vi "Code Point Substring.vi"(5 "End":i32, 7 "Start":i32, 11 "Constructor String Parser":T1) -> (3 "Substring":string)   [LabVIEW 2020, in "Stream.lvlib" / "URLPattern.lvclass"]
uses:
  URLPattern.lvclass
  Token Type.ctl
  Token.ctl
  URL Pattern Init.ctl
  Parser State.ctl
  Constructor String Parser.ctl
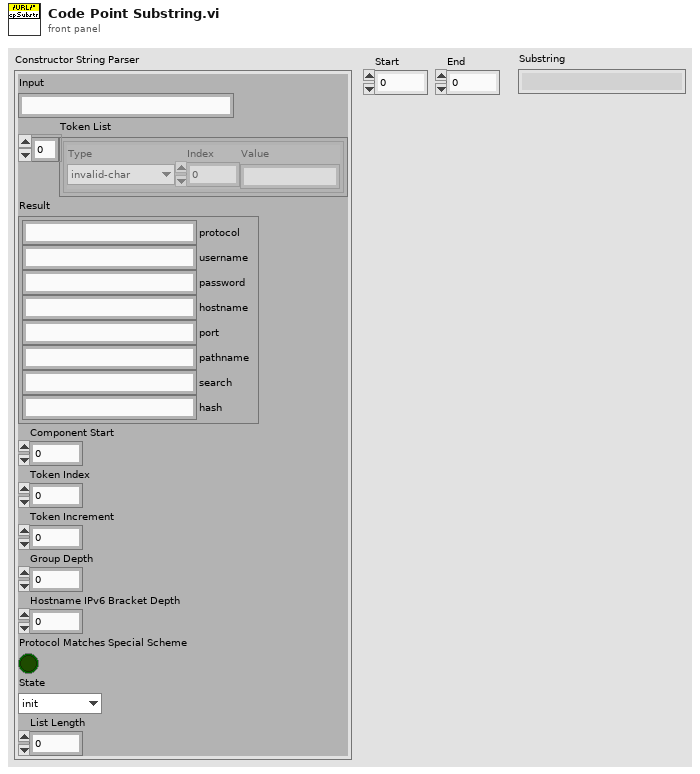
[diagram p1: front panel]
types:
  T1 = typedef "Stream.lvlib/URLPattern.lvclass/Constructor String Parser.ctl" = cluster{"Input":string, "Token List":T2[], "Result":T4, "Component Start":i32, "Token Index":i32, "Token Increment":i32, "Group Depth":i32, "Hostname IPv6 Bracket Depth":i32, "Protocol Matches Special Scheme":bool, "State":T5, "List Length":i32}
  T2 = typedef "Stream.lvlib/URLPattern.lvclass/Token.ctl" = cluster{"Type":T3, "Index":i32, "Value":string}
  T3 = typedef "Stream.lvlib/URLPattern.lvclass/Token Type.ctl" = enum16{"invalid-char", "open", "close", "regexp", "name", "char", "escaped-char", "other-modifier", "asterisk", "end"}
  T4 = typedef "Stream.lvlib/URLPattern.lvclass/URL Pattern Init.ctl" = cluster{"protocol":string, "username":string, "password":string, "hostname":string, "port":string, "pathname":string, "search":string, "hash":string}
  T5 = typedef "Stream.lvlib/URLPattern.lvclass/Parser State.ctl" = enum16{"init", "protocol", "authority", "username", "password", "hostname", "port", "pathname", "search", "hash", "done"}
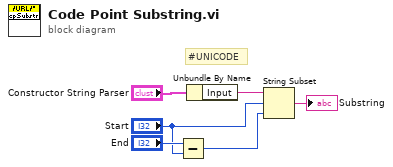
[diagram p0: block diagram]
diagram:
  # "#UNICODE"
  n1 = Subtract(x="End", y="Start") -> (x-y=w2:i32)
  n2 = Unbundle By Name("Constructor String Parser") -> ("Input"=w4:string)
  n3 = String Subset(string=w4, offset (0)="Start", length (rest)=w2) -> (substring=→"Substring":string)
